vi "Sensor Name Concatenate.vi"(10 "Array 2":string[](array[string]), 11 "Array":bool[](array[boolean])) -> (3 "String":string)   [LabVIEW 2021]
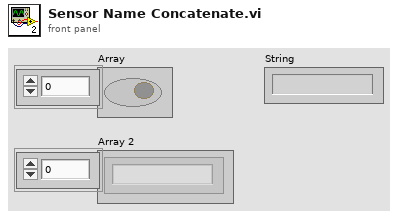
[diagram p1: front panel]
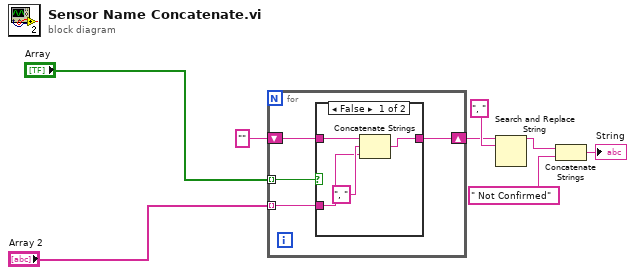
[diagram p0: block diagram]
diagram:
  n1 = for {
    tunnel: "Array 2" -> [w9] mode=indexing
    tunnel: "Array" -> [w12] mode=indexing
    shift-right: [w10] -> w4
    shift-left: "" -> [w11]
    n2 = case shown="False" w12 {
      tunnel: w11 -> [w15 w17]
      tunnel: [w16 w17] -> w10
      tunnel: w9 -> [w13 _]
      frame False {
        n3 = Concatenate Strings(w15, ", " ("string"), w13) -> (w16:string)
      }
      frame True {
      }
    }
  }
  n4 = Search and Replace String(input string=w4, search string=", " ("string")) -> (result string=w6:string)  [unwired: 6 in, 3 out]
  n5 = Concatenate Strings(w6, " Not Confirmed" ("string")) -> (→"String":string)
